vi "Read Histogram Bin Data Number.vi"(8 "error in (no error)":errorcluster, 9 "Measurement Type (0: Current)":i32(ring) items=["Current", "Limit", "Math", "Resistance", "Voltage"], 10 "Channel (1: Channel 1)":i32(ring)=1 items=["Channel 1"=1, "Channel 2"=2], 11 "VISA resource name":refnum<visa-resource-name>) -> (0 "error out":errorcluster, 1 "Lower Data Number Out of Bin":i32, 2 "Upper Data Number Out of Bin":i32, 3 "VISA resource name out":refnum<visa-resource-name>, 4 "Actual Bin Count":i32, 5 "Data Number In Bin":i32)   [LabVIEW 2012, in "Keysight B2980 Series.lvlib"]
doc: "Returns the number of data in each bin or out of bins range on Histogram view."
uses:
  Keysight B2980 Series.lvlib
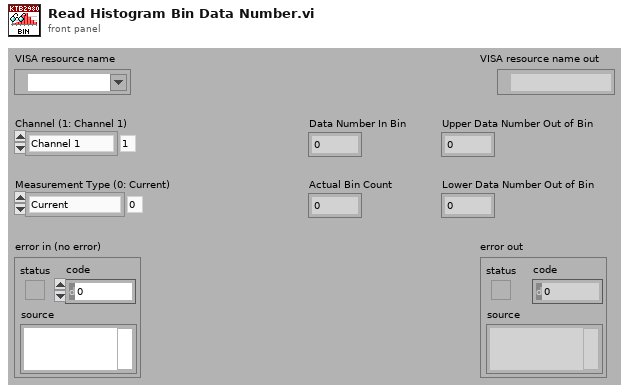
[diagram p1: front panel]
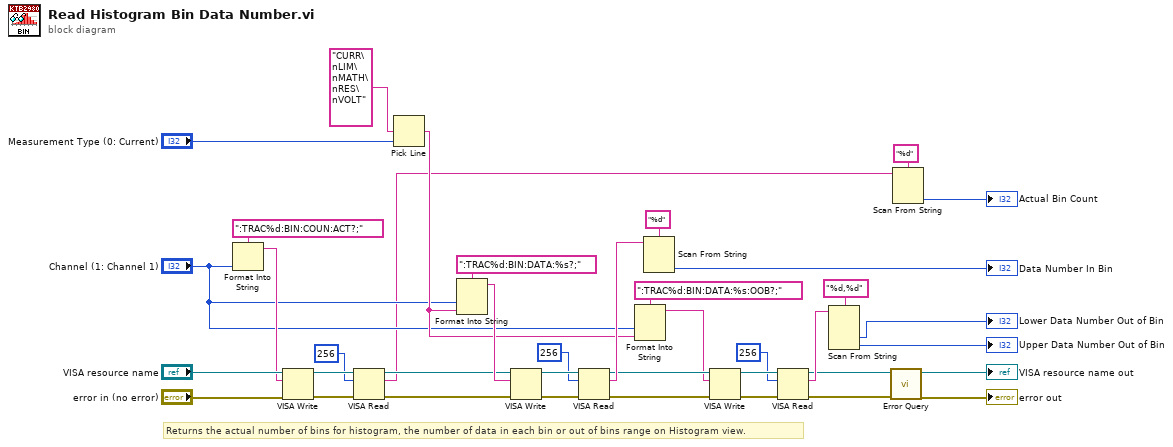
[diagram p0: block diagram]
diagram:
  # "Returns the actual number of bins for histogram, the number of data in each bin or out of bins range on Histogram view."
  n1 = Format Into String(format string=":TRAC%d:BIN:COUN:ACT?;", "Channel (1: Channel 1)") -> (resulting string=w3:string)  [unwired: 2 in, 1 out]
  n2 = VISA Write(VISA resource name="VISA resource name", write buffer=w3, error in (no error)="error in (no error)") -> (VISA resource name out=w12:refnum<visa-resource-name>, error out=w11:errorcluster)  [unwired: 1 out]
  n3 = VISA Read(VISA resource name=w12, byte count=u32 256, error in (no error)=w11) -> (VISA resource name out=w5:refnum<visa-resource-name>, read buffer=w1:string, error out=w4:errorcluster)  [unwired: 1 out]
  n4 = Pick Line(multi-line string="CURR\nLIM\nMATH\nRES\nVOLT", line index="Measurement Type (0: Current)") -> (output string=w26:string)  [unwired: 1 out]
  n5 = Format Into String(format string=":TRAC%d:BIN:DATA:%s?;", "Channel (1: Channel 1)", w26) -> (resulting string=w27:string)  [unwired: 2 in, 1 out]
  n6 = VISA Write(VISA resource name=w5, write buffer=w27, error in (no error)=w4) -> (VISA resource name out=w35:refnum<visa-resource-name>, error out=w34:errorcluster)  [unwired: 1 out]
  n7 = VISA Read(VISA resource name=w35, byte count=u32 256, error in (no error)=w34) -> (VISA resource name out=w22:refnum<visa-resource-name>, read buffer=w32:string, error out=w21:errorcluster)  [unwired: 1 out]
  n8 = Format Into String(format string=":TRAC%d:BIN:DATA:%s:OOB?;", "Channel (1: Channel 1)", w26) -> (resulting string=w14:string)  [unwired: 2 in, 1 out]
  n9 = Scan From String(format string="%d", input string=w32) -> (output 1=→"Data Number In Bin":i32)  [unwired: 2 in, 4 out]
  n10 = VISA Write(VISA resource name=w22, write buffer=w14, error in (no error)=w21) -> (VISA resource name out=w25:refnum<visa-resource-name>, error out=w24:errorcluster)  [unwired: 1 out]
  n11 = VISA Read(VISA resource name=w25, byte count=u32 256, error in (no error)=w24) -> (VISA resource name out=w16:refnum<visa-resource-name>, read buffer=w19:string, error out=w15:errorcluster)  [unwired: 1 out]
  n12 = Scan From String(format string="%d,%d", input string=w19) -> (output 1=→"Lower Data Number Out of Bin":i32, output 2=→"Upper Data Number Out of Bin":i32)  [unwired: 2 in, 5 out]
  n13 = call "Error Query.vi"("error in (no error)"=w15, "VISA resource name"=w16) -> ("error out"=→"error out":errorcluster, "VISA resource name out"=→"VISA resource name out":refnum<visa-resource-name>)  [unwired: 8 out]
  n14 = Scan From String(format string="%d", input string=w1) -> (output 1=→"Actual Bin Count":i32)  [unwired: 2 in, 4 out]
